vi "quadratic-roots_2.vi"() -> ()   [LabVIEW 2023]
panel:
  out "Boolean 4":bool
  out "Boolean 3":bool
  out "Boolean 2":bool
  out "Boolean":bool
  in  "Resolve":bool
  in  "stop":bool
  out "Root 2:":dbl
  out "Root 1:":dbl
  in  "C:":dbl
  in  "B:":dbl
  in  "A:":dbl
  # "Quadratic Roots Solver"
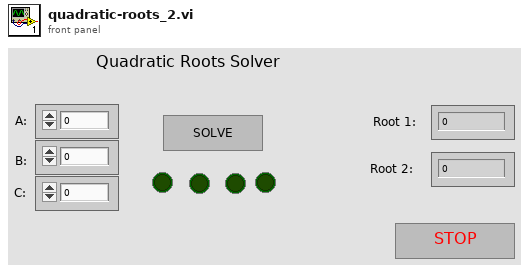
[diagram p1: front panel]
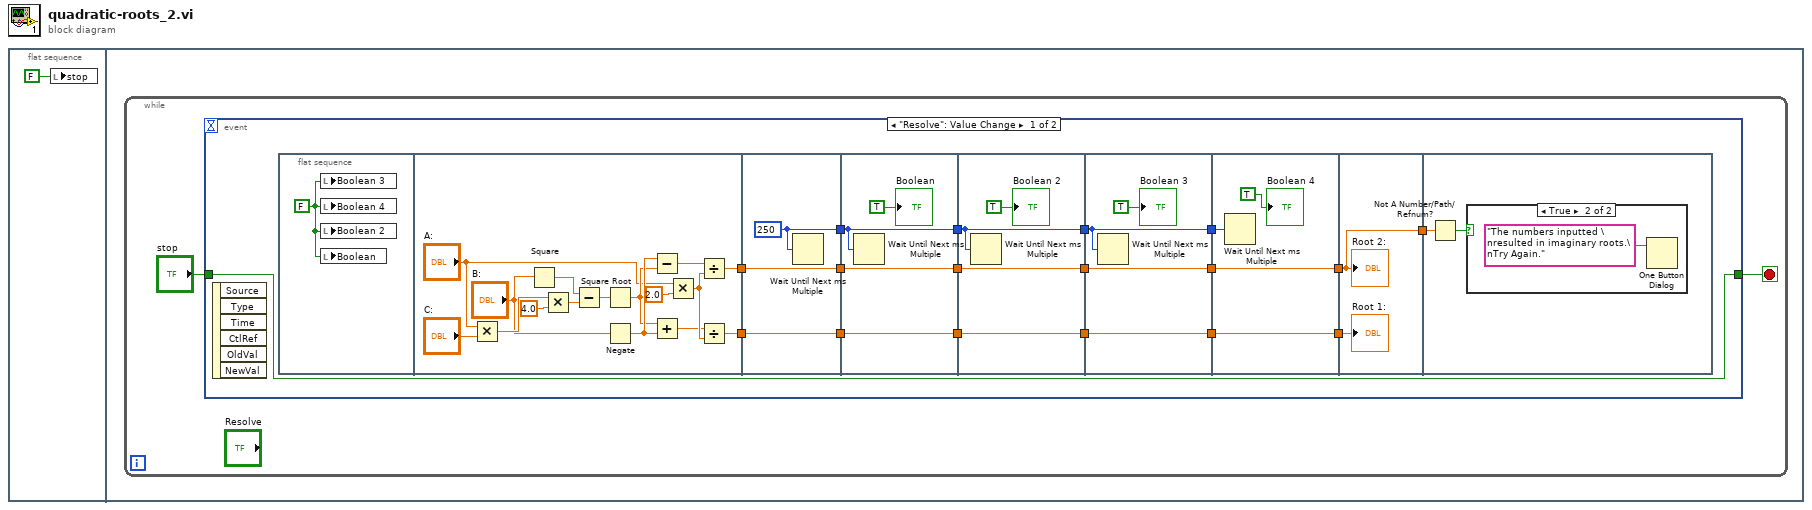
[diagram p0: block diagram]
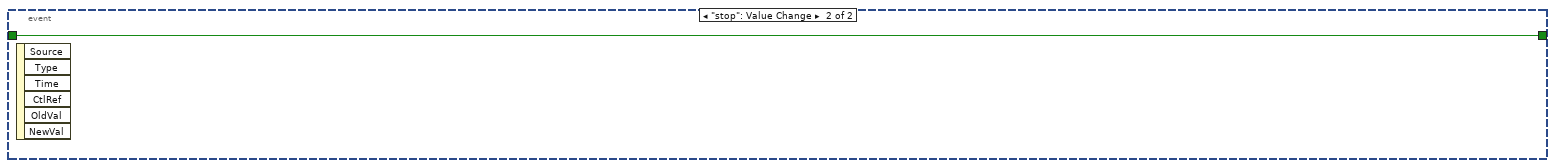
[diagram p3: hidden frame]
diagram:
  n1 = flat-sequence {
    frame #0 {
      n2 = local write "stop"(FALSE ("stop")) -> ()
    }
    frame #1 {
      n3 = while {
        stop <- w2 stop-if-true
        n4 = event shown="[0] \"Resolve\": Value Change" {
          selector: _ -> [_ _]
          dyn-events: _ -> [_ _]
          timeout: _ -> [_ _]
          tunnel: [w21 w63] -> w2
          tunnel: "stop" -> [w21 w63]
          event "Resolve": Value Change {
            n5 = event-data() -> ()  [unwired: 1 in, 6 out]
            n6 = flat-sequence {
              tunnel: [w24] -> w14
              tunnel: [w23] -> w12
              tunnel: w14 -> [w41]
              tunnel: [w41] -> w13
              tunnel: w12 -> [w40]
              tunnel: [w40] -> w11
              tunnel: [w39] -> w7
              tunnel: w13 -> [w45]
              tunnel: w11 -> [w44]
              tunnel: [w45] -> w20
              tunnel: [w44] -> w19
              tunnel: w7 -> [w42]
              tunnel: [w42] -> w6
              tunnel: w20 -> [w49]
              tunnel: [w49] -> w18
              tunnel: w19 -> [w48]
              tunnel: [w48] -> w16
              tunnel: w6 -> [w46]
              tunnel: [w46] -> w5
              tunnel: w18 -> [w53]
              tunnel: [w53] -> w17
              tunnel: w16 -> [w52]
              tunnel: [w52] -> w15
              tunnel: w5 -> [w50]
              tunnel: [w50] -> w4
              tunnel: w17 -> [w57]
              tunnel: w15 -> [w56]
              tunnel: [w57] -> w10
              tunnel: [w56] -> w9
              tunnel: w4 -> [w54]
              tunnel: w10 -> [w58]
              tunnel: w9 -> [w59]
              tunnel: [w59] -> w8
              tunnel: w8 -> [w60]
              frame #0 {
                w22 = FALSE ("Boolean 3")
                n7 = local write "Boolean 3"(w22) -> ()
                n8 = local write "Boolean 4"(w22) -> ()
                n9 = local write "Boolean 2"(w22) -> ()
                n10 = local write "Boolean"(w22) -> ()
              }
              frame #1 {
                n11 = Multiply(x="A:", y="C:") -> (x*y=w37:dbl)
                n12 = Square(x="B:") -> (x^2=w35:dbl)
                n13 = Multiply(x=w37, y=4.0) -> (x*y=w34:dbl)
                n14 = Subtract(x=w35, y=w34) -> (x-y=w33:dbl)
                n15 = Square Root(x=w33) -> (sqrt(x)=w30:dbl)
                n16 = Negate(x="B:") -> (-x=w31:dbl)
                n17 = Subtract(x=w31, y=w30) -> (x-y=w27:dbl)
                n18 = Add(x=w30, y=w31) -> (x+y=w25:dbl)
                n19 = Multiply(x="A:", y=2.0) -> (x*y=w26:dbl)
                n20 = Divide(x=w27, y=w26) -> (x/y=w23:dbl)
                n21 = Divide(x=w25, y=w26) -> (x/y=w24:dbl)
              }
              frame #2 {
                w39 = u32 250 ("millisecond multiple")
                n22 = Wait Until Next ms Multiple(millisecond multiple=w39) -> ()  [unwired: 1 out]
              }
              frame #3 {
                n23 = Wait Until Next ms Multiple(millisecond multiple=w42) -> ()  [unwired: 1 out]
                "Boolean" <- TRUE ("Boolean")
              }
              frame #4 {
                n24 = Wait Until Next ms Multiple(millisecond multiple=w46) -> ()  [unwired: 1 out]
                "Boolean 2" <- TRUE ("Boolean 2")
              }
              frame #5 {
                n25 = Wait Until Next ms Multiple(millisecond multiple=w50) -> ()  [unwired: 1 out]
                "Boolean 3" <- TRUE ("Boolean 3")
              }
              frame #6 {
                n26 = Wait Until Next ms Multiple(millisecond multiple=w54) -> ()  [unwired: 1 out]
                "Boolean 4" <- TRUE ("Boolean 4")
              }
              frame #7 {
                "Root 2:" <- w59
                "Root 1:" <- w58
              }
              frame #8 {
                n27 = Not A Number/Path/Refnum?(number/path/refnum=w60) -> (NaN/Path/Refnum?=w61:bool)
                n28 = case shown="True" w61 {
                  frame False {
                  }
                  frame True {
                    n29 = One Button Dialog(message="The numbers inputted \nresulted in imaginary roots.\nTry Again.") -> ()  [unwired: 1 in, 1 out]
                  }
                }
              }
            }
          }
          event "stop": Value Change {
            n30 = event-data() -> ()  [unwired: 1 in, 6 out]
          }
        }
      }
    }
  }
